vi "DequeueMessage.vi"(8 "error in (no error)":errorcluster, 11 "MessageQueue":refnum<queue>) -> (0 "error out":errorcluster, 1 "MessageData":variant, 2 "Message":string, 3 "dupMessageQueue":refnum<queue>)   [LabVIEW 2015]
doc: "Nimmt die erste Nachricht aus der Queue."
uses:
  TypeDefs/MessageCluster.ctl
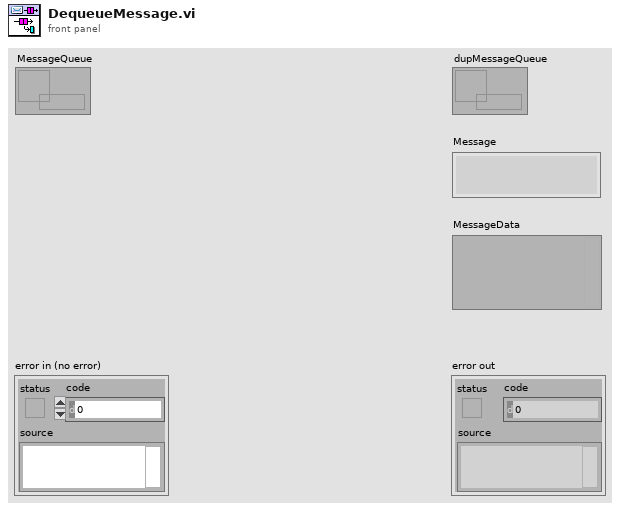
[diagram p1: front panel]
types:
  T1 = typedef "MessageCluster.ctl" = cluster{"Message":string, "MessageData":variant}
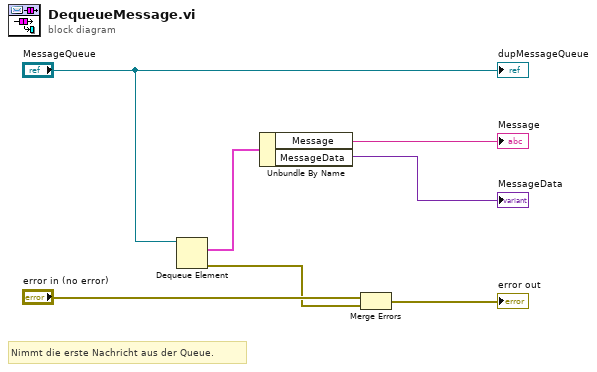
[diagram p0: block diagram]
diagram:
  # "Nimmt die erste Nachricht aus der Queue."
  n1 = Dequeue Element(queue="MessageQueue") -> (element=w4:T1, error out=w1:errorcluster)  [unwired: 2 in, 2 out]
  n2 = Unbundle By Name(w4) -> ("Message"=→"Message":string, "MessageData"=→"MessageData":variant)
  n3 = Merge Errors("error in (no error)", w1) -> (→"error out":errorcluster)
  "dupMessageQueue" <- "MessageQueue"
